vi "initialize NI card.vi"(7 "do waveforms":T5[](array[typedef]), 11 "error in":errorcluster) -> (4 "main trigger":refnum<k21>, 15 "error out":errorcluster)   [LabVIEW 2015]
uses:
  type def/NI card channels.ctl
  type def/do waveform.ctl
  type def/basic params.ctl
  type def/advanced params.ctl
  type def/PXI control.ctl
  <instrlib>/niScope/Controls/niScope trigger source digital.ctl
  <instrlib>/niScope/Controls/niScope trigger slope.ctl
  <vilib>/DAQmx/write.llb/DAQmx Write (Digital 1D U32 1Chan NSamp).vi
  global variables/params.vi
  <instrlib>/niScope/Configure/Trigger/niScope Configure Trigger Digital.vi
  <vilib>/DAQmx/create/channels.llb/DAQmx Create Channel (CO-Pulse Generation-Time).vi
  <vilib>/DAQmx/configure/timing.llb/DAQmx Timing (Implicit).vi
  <vilib>/DAQmx/configure/trigger.llb/DAQmx Start Trigger (None).vi
  <vilib>/DAQmx/configure/trigger.llb/DAQmx Start Trigger (Digital Edge).vi
  <vilib>/DAQmx/create/channels.llb/DAQmx Create Channel (CO-Pulse Generation-Frequency).vi
  <vilib>/DAQmx/create/channels.llb/DAQmx Create Channel (DO-Digital Output).vi
  <vilib>/DAQmx/configure/timing.llb/DAQmx Timing (Sample Clock).vi
  <vilib>/DAQmx/miscellaneous.llb/DAQmx Fill In Error Info.vi
  <resource>/objmgr/daqmx.rc
panel:
  in  "PXI channel":T1={"Vertical Range (V)"=1.0, "Min Sample Rate"=2208791.906743315, "# of Channels"=1, "Min Record Length"=560, "Number Of Records"=10000, "Trigger Position(%)"=0.0, "act Record Length"=1000, "trigger source"="VAL_EXTERNAL", "PMT2 # of Channels"=1} {"PMT2 # of Channels" min=1 max=8 step=1; "act Record Length" min=0 max=100 format="%#.3g"; "Trigger Position(%)" min=0.0 max=1000000.0 step=1.0 format="%#.3p"; "Number Of Records" min=0 max=10000 step=1 format="%#.3g"; "Min Record Length" min=1 max=8 step=1; "# of Channels" min=1 max=8 step=1; "Min Sample Rate" min=0.0 max=100000000.0 format="%#.3p"; "Vertical Range (V)" min=0.0 max=10.0 format="%#.3g"}
  in  "advanced params":T3={"x flyback time(%)"=40.0, "signal offset"=0, "frame time(s)"=0.0, "fetch # per frame"=1, "galvo sampling rate"=500000} {"galvo sampling rate" min=10000 max=200000 step=1; "fetch # per frame" min=1 max=100 step=1 format="%#.3g"; "frame time(s)" min=0.0 max=100.0 step=0.1 format="%#.3g"; "signal offset" max=10000 format="%#.3g"; "x flyback time(%)" min=0.0 max=50.0 format="%#.3g"}
  in  "basic params":T4={"X pixel #"=200, "X pixel size(um)"=1.0, "Y pixel #"=200, "Y pixel size(um)"=10.0, "line rate(Hz)"=1.0, "stage scan?"=FALSE} {"line rate(Hz)" min=1.0 max=2000.0 format="%#.3g"; "X pixel size(um)" min=0.0 max=10.0 format="%#.3g"; "X pixel #" min=2 max=20480 step=2 format="%#.3g"; "Y pixel size(um)" min=0.0 max=10.0 format="%#.3g"; "Y pixel #" min=2 max=204800 step=2 format="%#.3g"}
  in  "do":T6=[{"signal"="x galvo", "DAQmx Physical Channel"="Dev1/ao0", "max"=10.0, "min"=-10.0, "DAQmx Terminal"="", "start trigger"="", "ClockSource"="", "Scaling Factor"=1.0, "Notes"=""}, {"signal"="y galvo", "DAQmx Physical Channel"="Dev1/ao1", "max"=10.0, "min"=-10.0, "DAQmx Terminal"="", "start trigger"="", "ClockSource"="", "Scaling Factor"=1.0, "Notes"=""}]
  in  "triggers":T6=[{"signal"="x galvo", "DAQmx Physical Channel"="Dev1/ao0", "max"=10.0, "min"=-10.0, "DAQmx Terminal"="", "start trigger"="", "ClockSource"="", "Scaling Factor"=1.0, "Notes"=""}, {"signal"="y galvo", "DAQmx Physical Channel"="Dev1/ao1", "max"=10.0, "min"=-10.0, "DAQmx Terminal"="", "start trigger"="", "ClockSource"="", "Scaling Factor"=1.0, "Notes"=""}]
  in  "NI card channels":T6=[{"signal"="x galvo", "DAQmx Physical Channel"="Dev1/ao0", "max"=10.0, "min"=-10.0, "DAQmx Terminal"="", "start trigger"="", "ClockSource"="", "Scaling Factor"=1.0, "Notes"=""}, {"signal"="y galvo", "DAQmx Physical Channel"="Dev1/ao1", "max"=10.0, "min"=-10.0, "DAQmx Terminal"="", "start trigger"="", "ClockSource"="", "Scaling Factor"=1.0, "Notes"=""}]
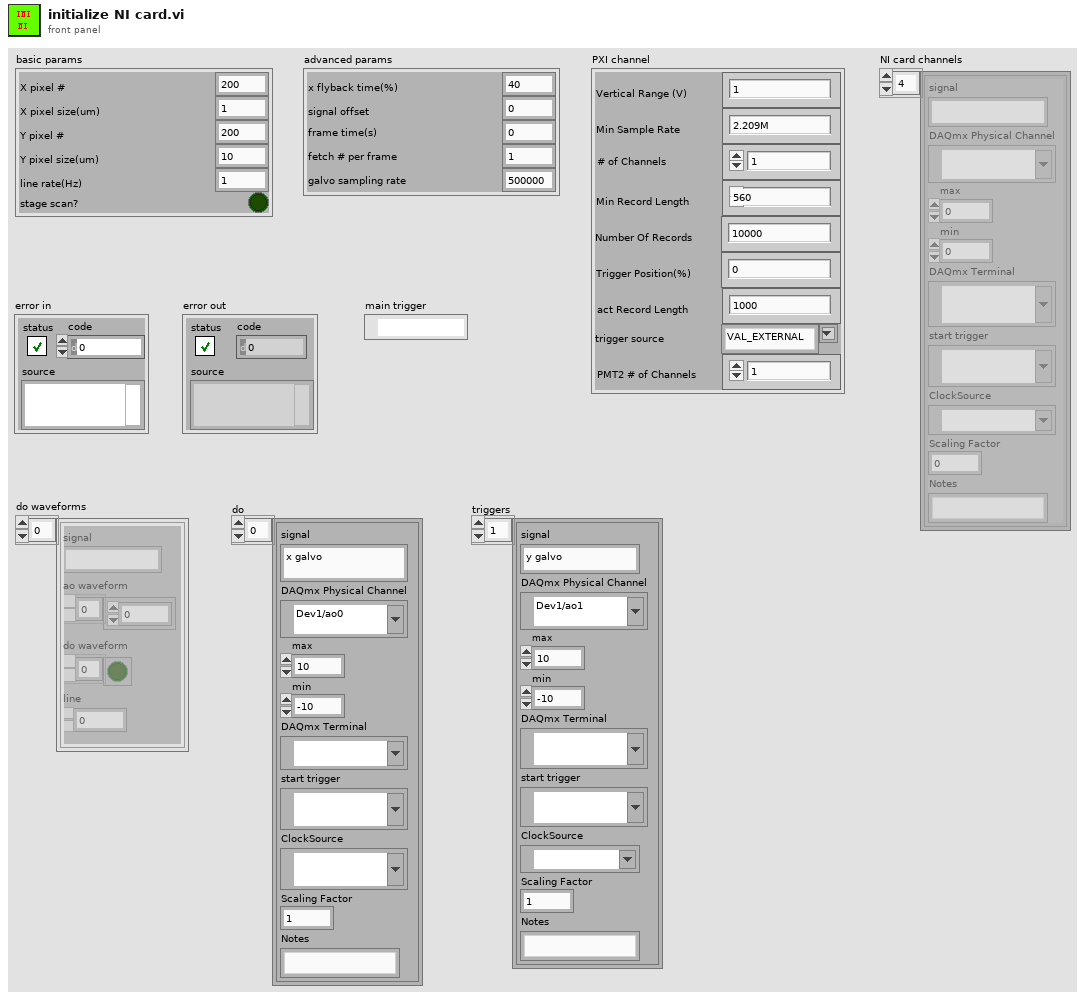
[diagram p1: front panel]
types:
  T1 = typedef "PXI control.ctl" = cluster{"Vertical Range (V)":dbl, "Min Sample Rate":dbl, "# of Channels":u8, "Min Record Length":i32, "Number Of Records":i32, "Trigger Position(%)":dbl, "act Record Length":i32, "trigger source":T2, "PMT2 # of Channels":u8}
  T2 = typedef "niScope trigger source digital.ctl" = string
  T3 = typedef "advanced params.ctl" = cluster{"x flyback time(%)":dbl, "signal offset":u16, "frame time(s)":dbl, "fetch # per frame":u16, "galvo sampling rate":u32}
  T4 = typedef "basic params.ctl" = cluster{"X pixel #":u32, "X pixel size(um)":dbl, "Y pixel #":u32, "Y pixel size(um)":dbl, "line rate(Hz)":dbl, "stage scan?":bool}
  T5 = typedef "do waveform.ctl" = cluster{"signal":string, "ao waveform":dbl[], "do waveform":bool[], "line":u8}
  T6 = typedef "NI card channels.ctl" = cluster{"signal":string, "DAQmx Physical Channel":tag, "max":dbl, "min":dbl, "DAQmx Terminal":tag, "start trigger":tag, "ClockSource":tag, "Scaling Factor":dbl, "Notes":string}[]
  T7 = cluster{"signal":string, "DAQmx Physical Channel":tag, "max":dbl, "min":dbl, "DAQmx Terminal":tag, "start trigger":string, "ClockSource":tag, "Scaling Factor":dbl, "Notes":string}[]
  T8 = typedef "niScope trigger slope.ctl" = i32
  T9 = typedef "NI tasks.ctl" = cluster{"frame trigger":refnum<k21>, "do":refnum<k21>, "digital galvo clock":refnum<k21>, "PMT in":refnum<k15>, "PMT2 in":refnum<k15>}
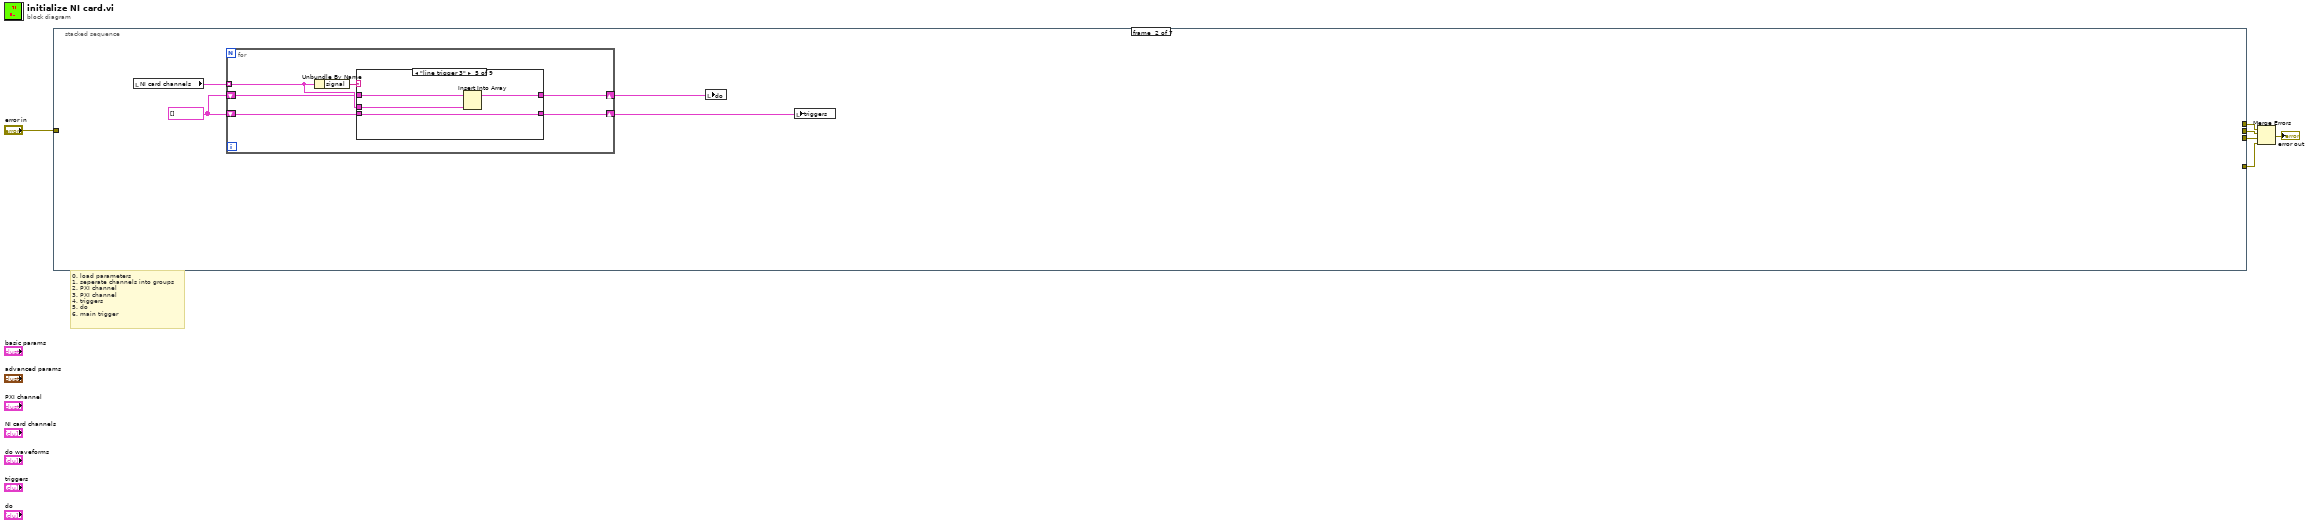
[diagram p0: block diagram]
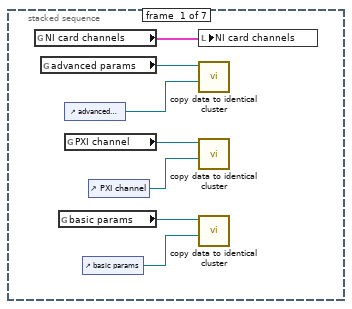
[diagram p2: hidden frame]
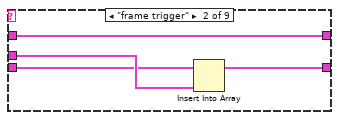
[diagram p4: hidden frame]
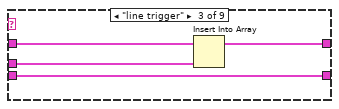
[diagram p5: hidden frame]
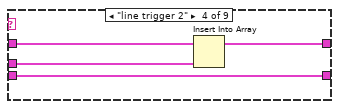
[diagram p6: hidden frame]
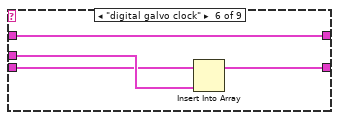
[diagram p7: hidden frame]
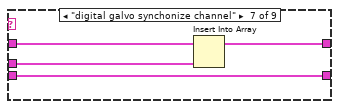
[diagram p8: hidden frame]
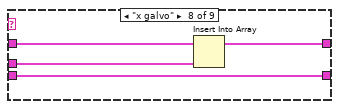
[diagram p9: hidden frame]
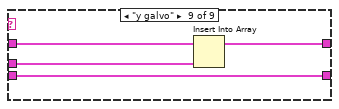
[diagram p10: hidden frame]
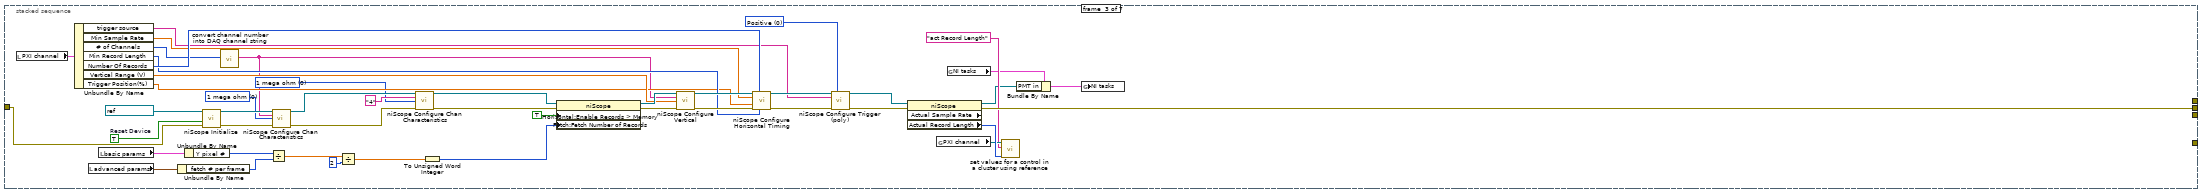
[diagram p11: hidden frame]
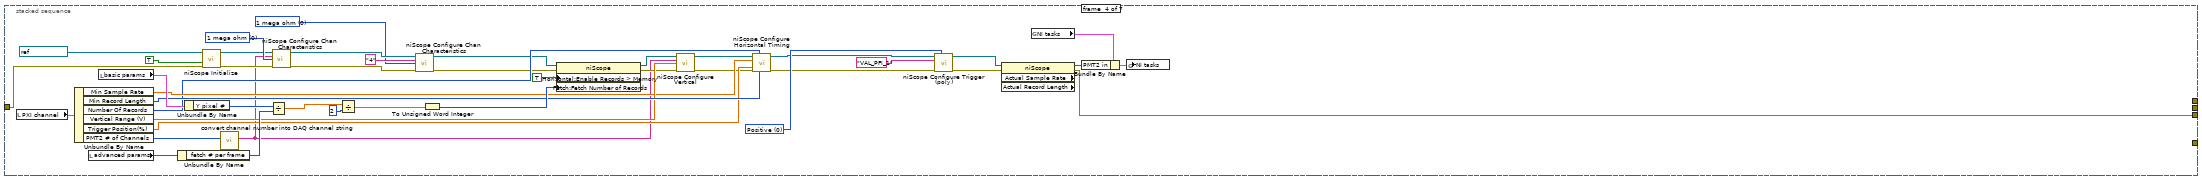
[diagram p12: hidden frame]
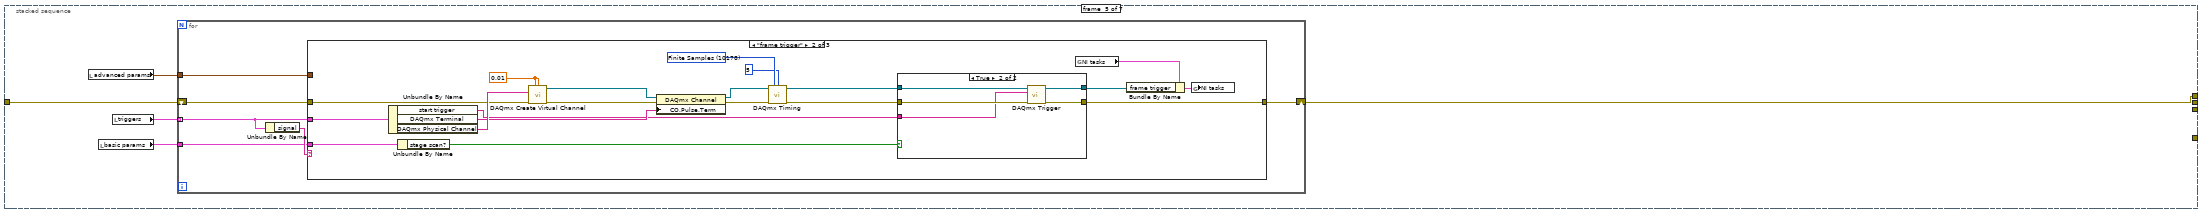
[diagram p13: hidden frame]
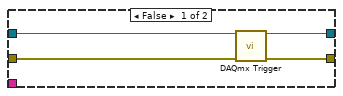
[diagram p15: hidden frame]
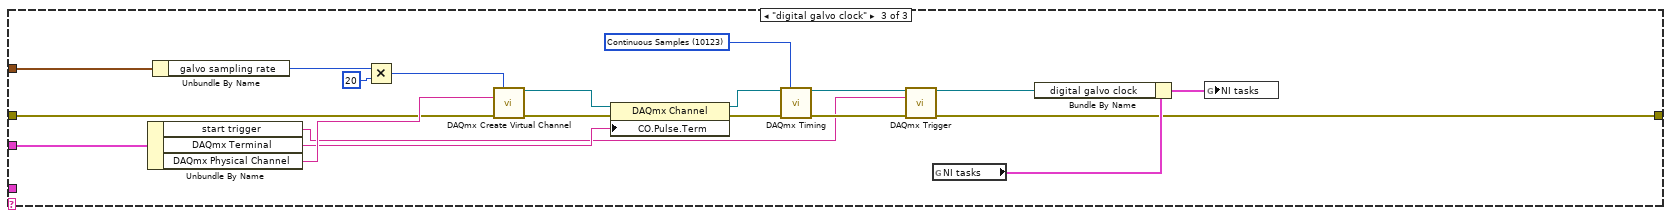
[diagram p16: hidden frame]
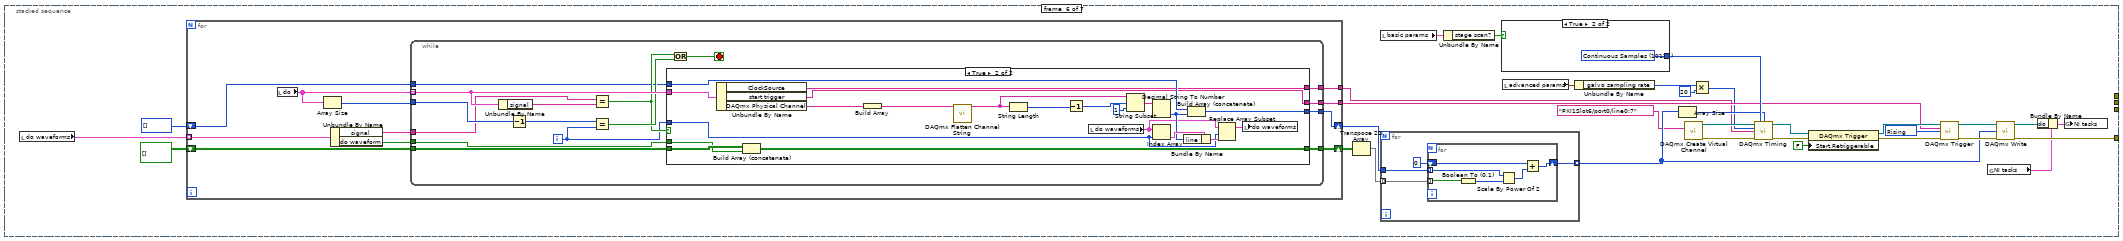
[diagram p17: hidden frame]
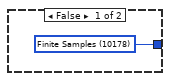
[diagram p18: hidden frame]
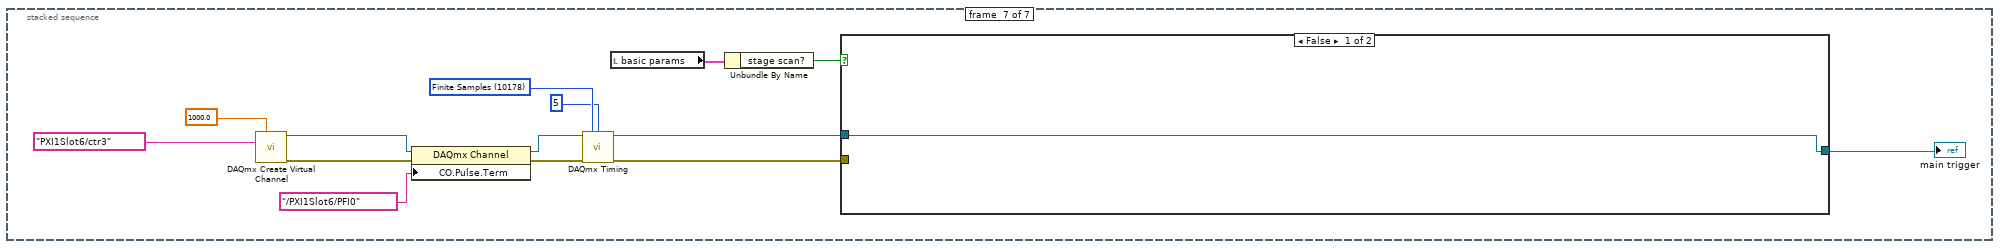
[diagram p20: hidden frame]
diagram:
  # "0. load parameters\n1. seperate channels into groups\n2. PXI channel\n3. PXI channel\n4. triggers\n5. do\n6. main trigger"
  n1 = stacked-sequence {
    tunnel: "error in" -> [_ _ w97 w118 w150 _ _]
    tunnel: [_ _ w87 _ _ _ _] -> w2
    tunnel: [_ _ _ _ w149 _ _] -> w3
    tunnel: [_ _ _ _ _ w227 _] -> w4
    tunnel: [_ _ _ w114 _ _ _] -> w1
    frame #0 {
      n2 = global read "params.vi" "NI card channels"() -> (w12:T6)
      n3 = global read "params.vi" "advanced params"() -> (w13:refnum<vi>)
      n4 = global read "params.vi" "basic params"() -> (w11:refnum<vi>)
      n5 = control-ref of="advanced params"() -> (w8:refnum<vi>)
      n6 = global read "params.vi" "PXI channel"() -> (w10:refnum<vi>)
      n7 = control-ref of="basic params"() -> (w9:refnum<vi>)
      n8 = control-ref of="PXI channel"() -> (w7:refnum<vi>)
      n9 = local write "NI card channels"(w12) -> ()
      n10 = call "copy data to identical cluster.vi"("Guest Clust Refnum"=w8, "Host Clust Refnum"=w13) -> ()  [unwired: 10 in]
      n11 = call "copy data to identical cluster.vi"("Guest Clust Refnum"=w7, "Host Clust Refnum"=w10) -> ()  [unwired: 10 in]
      n12 = call "copy data to identical cluster.vi"("Guest Clust Refnum"=w9, "Host Clust Refnum"=w11) -> ()  [unwired: 10 in]
    }
    frame #1 {
      w14 = T7 []
      n13 = local read "NI card channels"() -> (w17:T6)
      n14 = for {
        tunnel: w17 -> [w22] mode=indexing
        shift-right: [w21] -> w16
        shift-left: w14 -> [w18]
        shift-right: [w20] -> w15
        shift-left: w14 -> [w19]
        n15 = Unbundle By Name(w22) -> ("signal"=w23:string)
        n16 = case shown="\"line trigger 3\"" w23 {
          tunnel: w22 -> [_ w29 w33 w37 w41 w45 w49 w53 w57]
          tunnel: [w25 w27 w30 w34 w38 w44 w48 w50 w56] -> w21
          tunnel: w18 -> [w25 w26 w30 w34 w38 w43 w48 w50 w56]
          tunnel: [w24 w28 w32 w36 w40 w42 w46 w52 w54] -> w20
          tunnel: w19 -> [w24 w28 w31 w35 w39 w42 w47 w51 w55]
          frame "False", Default {
          }
          frame "frame trigger" {
            n17 = Insert Into Array(array=w26, new element=w29) -> (w27:T7)  [unwired: 1 in]
          }
          frame "line trigger" {
            n18 = Insert Into Array(array=w31, new element=w33) -> (w32:T7)  [unwired: 1 in]
          }
          frame "line trigger 2" {
            n19 = Insert Into Array(array=w35, new element=w37) -> (w36:T7)  [unwired: 1 in]
          }
          frame "line trigger 3" {
            n20 = Insert Into Array(array=w39, new element=w41) -> (w40:T7)  [unwired: 1 in]
          }
          frame "digital galvo clock" {
            n21 = Insert Into Array(array=w43, new element=w45) -> (w44:T7)  [unwired: 1 in]
          }
          frame "digital galvo synchonize channel" {
            n22 = Insert Into Array(array=w47, new element=w49) -> (w46:T7)  [unwired: 1 in]
          }
          frame "x galvo" {
            n23 = Insert Into Array(array=w51, new element=w53) -> (w52:T7)  [unwired: 1 in]
          }
          frame "y galvo" {
            n24 = Insert Into Array(array=w55, new element=w57) -> (w54:T7)  [unwired: 1 in]
          }
        }
      }
      n25 = local write "do"(w15) -> ()
      n26 = local write "triggers"(w16) -> ()
    }
    frame #2 {
      w58 = u32 0 items=["1 mega ohm"=0, "50 ohms"=2] ("input impedance")
      w66 = u32 0 items=["1 mega ohm"=0, "50 ohms"=2] ("input impedance")
      w77 = T8 0 items=["Positive", "Negative"] ("trigger slope")
      w103 = TRUE  # Reset Device
      n27 = local read "PXI channel"() -> (w96:T1)
      n28 = Unbundle By Name(w96) -> ("trigger source"=w69:T2, "Min Sample Rate"=w89:dbl, "# of Channels"=w70:u8, "Min Record Length"=w86:i32, "Number Of Records"=w98:i32, "Vertical Range (V)"=w68:dbl, "Trigger Position(%)"=w67:dbl)
      n29 = local read "advanced params"() -> (w95:T3)
      n30 = local read "basic params"() -> (w94:T4)
      n31 = Unbundle By Name(w95) -> ("fetch # per frame"=w76:u16)
      n32 = Unbundle By Name(w94) -> ("Y pixel #"=w91:u32)
      n33 = call <instrlib>:"niScope Initialize.vi"("resource name"=refnum<k15> "PXI1Slot2", "reset device"=w103, "error in"=w97) -> ("instrument handle"=w85:refnum<k15>, "error out"=w84:errorcluster)  [unwired: 11 in]
      n34 = call "convert channel number into DAQ channel string.vi"("Numeric"=w70) -> ("String"=w65:string)  [unwired: 10 in]
      n35 = Divide(x=w91, y=w76) -> (x/y=w74:dbl)
      n36 = call <instrlib>:"niScope Configure Chan Characteristics.vi"("instrument handle"=w85, "channels"=w65, "input impedance"=w66, "error in"=w84) -> ("instrument handle out"=w61:refnum<k15>, "error out"=w60:errorcluster)  [unwired: 10 in]
      n37 = Divide(x=w74, y=2) -> (x/y=w73:dbl)
      n38 = call <instrlib>:"niScope Configure Chan Characteristics.vi"("instrument handle"=w61, "channels"="4", "input impedance"=w58, "error in"=w60) -> ("instrument handle out"=w63:refnum<k15>, "error out"=w62:errorcluster)  [unwired: 10 in]
      n39 = To Unsigned Word Integer(number=w73) -> (unsigned 16bit integer=w72:u16)
      n40 = property class="niScope"(reference=w63, error in=w62, "Horizontal:Enable Records > Memory"=TRUE ("Allow More Records\nthan Available Memory?"), "Fetch:Fetch Number of Records"=w72) -> (reference out=w93:refnum<k15>, error out=w92:errorcluster)
      n41 = call <instrlib>:"niScope Configure Vertical.vi"("instrument handle"=w93, "channels"=w65, "vertical range"=w68, "error in"=w92) -> ("instrument handle out"=w101:refnum<k15>, "error out"=w100:errorcluster)  [unwired: 10 in]
      n42 = call <instrlib>:"niScope Configure Horizontal Timing.vi"("instrument handle"=w101, "number of records"=w98, "min sample rate"=w89, "reference position"=w67, "error in"=w100, "min record length"=w86) -> ("instrument handle out"=w71:refnum<k15>, "error out"=w99:errorcluster)  [unwired: 8 in]
      n43 = call-poly <instrlib>:"niScope Configure Trigger (poly).vi"("instrument handle"=w71, "trigger slope"=w77, "trigger source"=w69, "error in"=w99) -> ("instrument handle out"=w90:refnum<k15>, "error out"=w88:errorcluster)  [unwired: 10 in]
      n44 = property class="niScope" props=["Actual Sample Rate", "Actual Record Length"](reference=w90, error in=w88) -> (reference out=w80:refnum<k15>, error out=w87:errorcluster, "Actual Record Length"=w83:i32)  [unwired: 1 out]
      n45 = global read "params.vi" "PXI channel"() -> (w82:refnum<vi>)
      n46 = global read "params.vi" "NI tasks"() -> (w79:T9)
      n47 = call "set values for a control in a cluster using reference.vi"("value"=w83, "name"="act Record Length", "Clust Refnum"=w82) -> ()  [unwired: 9 in]
      n48 = Bundle By Name(cluster=w79, "PMT in"=w80) -> (w78:T9)
      n49 = global write "params.vi" "NI tasks"(w78) -> ()
    }
    frame #3 {
      w104 = u32 0 items=["1 mega ohm"=0, "50 ohms"=2] ("input impedance")
      w133 = T8 0 items=["Positive", "Negative"] ("trigger slope")
      w123 = u32 0 items=["1 mega ohm"=0, "50 ohms"=2] ("input impedance")
      n50 = local read "PXI channel"() -> (w127:T1)
      n51 = Unbundle By Name(w127) -> ("Min Sample Rate"=w135:dbl, "Min Record Length"=w138:i32, "Number Of Records"=w134:i32, "Vertical Range (V)"=w137:dbl, "Trigger Position(%)"=w136:dbl, "PMT2 # of Channels"=w111:u8)
      n52 = local read "advanced params"() -> (w143:T3)
      n53 = local read "basic params"() -> (w145:T4)
      n54 = Unbundle By Name(w143) -> ("fetch # per frame"=w142:u16)
      n55 = Unbundle By Name(w145) -> ("Y pixel #"=w146:u32)
      n56 = call <instrlib>:"niScope Initialize.vi"("resource name"=refnum<k15> "PXI1Slot3", "reset device"=TRUE, "error in"=w118) -> ("instrument handle"=w119:refnum<k15>, "error out"=w120:errorcluster)  [unwired: 11 in]
      n57 = call "convert channel number into DAQ channel string.vi"("Numeric"=w111) -> ("String"=w110:string)  [unwired: 10 in]
      n58 = Divide(x=w146, y=w142) -> (x/y=w140:dbl)
      n59 = call <instrlib>:"niScope Configure Chan Characteristics.vi"("instrument handle"=w119, "channels"=w110, "input impedance"=w123, "error in"=w120) -> ("instrument handle out"=w109:refnum<k15>, "error out"=w108:errorcluster)  [unwired: 10 in]
      n60 = Divide(x=w140, y=2) -> (x/y=w139:dbl)
      n61 = call <instrlib>:"niScope Configure Chan Characteristics.vi"("instrument handle"=w109, "channels"="4", "input impedance"=w104, "error in"=w108) -> ("instrument handle out"=w107:refnum<k15>, "error out"=w106:errorcluster)  [unwired: 10 in]
      n62 = To Unsigned Word Integer(number=w139) -> (unsigned 16bit integer=w144:u16)
      n63 = property class="niScope"(reference=w107, error in=w106, "Horizontal:Enable Records > Memory"=TRUE, "Fetch:Fetch Number of Records"=w144) -> (reference out=w125:refnum<k15>, error out=w126:errorcluster)
      n64 = call <instrlib>:"niScope Configure Vertical.vi"("instrument handle"=w125, "channels"=w110, "vertical range"=w137, "error in"=w126) -> ("instrument handle out"=w129:refnum<k15>, "error out"=w130:errorcluster)  [unwired: 10 in]
      n65 = call <instrlib>:"niScope Configure Horizontal Timing.vi"("instrument handle"=w129, "number of records"=w134, "min sample rate"=w135, "reference position"=w136, "error in"=w130, "min record length"=w138) -> ("instrument handle out"=w128:refnum<k15>, "error out"=w131:errorcluster)  [unwired: 8 in]
      n66 = call-poly <instrlib>:"niScope Configure Trigger (poly).vi"("instrument handle"=w128, "trigger slope"=w133, "trigger source"=T2 "VAL_PFI_1", "error in"=w131) -> ("instrument handle out"=w113:refnum<k15>, "error out"=w115:errorcluster)  [unwired: 10 in]
      n67 = property class="niScope" props=["Actual Sample Rate", "Actual Record Length"](reference=w113, error in=w115) -> (reference out=w112:refnum<k15>, error out=w114:errorcluster)  [unwired: 2 out]
      n68 = global read "params.vi" "NI tasks"() -> (w117:T9)
      n69 = Bundle By Name(cluster=w117, "PMT2 in"=w112) -> (w116:T9)
      n70 = global write "params.vi" "NI tasks"(w116) -> ()
    }
    frame #4 {
      n71 = local read "advanced params"() -> (w147:T3)
      n72 = local read "basic params"() -> (w148:T4)
      n73 = local read "triggers"() -> (w151:T6)
      n74 = for {
        tunnel: w151 -> [w156] mode=indexing
        shift-right: [w155] -> w149
        shift-left: w150 -> [w154]
        tunnel: w148 -> [w153]
        tunnel: w147 -> [w152]
        n75 = Unbundle By Name(w156) -> ("signal"=w157:string)
        n76 = case shown="\"frame trigger\"" w157 {
          tunnel: w156 -> [_ w178 w207]
          tunnel: w154 -> [w158 w170 w200]
          tunnel: [w158 w162 w196] -> w155
          tunnel: w153 -> [_ w159 _]
          tunnel: w152 -> [_ _ w192]
          frame "False", Default {
          }
          frame "frame trigger" {
            w167 = 0.01 ("high time")
            w171 = 10178 items=["Finite Samples"=10178, "Continuous Samples"=10123, "Hardware Timed Single Point"=12522] ("sample mode")
            n77 = Unbundle By Name(w178) -> ("start trigger"=w160:tag, "DAQmx Terminal"=w174:tag, "DAQmx Physical Channel"=w175:tag)
            n78 = Unbundle By Name(w159) -> ("stage scan?"=w161:bool)
            n79 = call-poly <vilib>:"DAQmx Create Virtual Channel.vi"("high time"=w167, "low time"=w167, "counter"=w175, "error in"=w170) -> ("task out"=w176:refnum<k21>, "error out"=w177:errorcluster)  [unwired: 10 in]
            n80 = property class="DAQmx Channel"(reference=w176, error in=w177, "CO.Pulse.Term"=w174) -> (reference out=w173:refnum<k21>, error out=w172:errorcluster)
            n81 = call-poly <vilib>:"DAQmx Timing.vi"("task/channels in"=w173, "sample mode"=w171, "samples per channel"=5, "error in"=w172) -> ("task out"=w165:refnum<k21>, "error out"=w163:errorcluster)  [unwired: 10 in]
            n82 = case shown="True" w161 {
              tunnel: w165 -> [w182 w187]
              tunnel: [w181 w186] -> w164
              tunnel: w163 -> [w180 w185]
              tunnel: [w179 w184] -> w162
              tunnel: w160 -> [_ w183]
              frame False {
                n83 = call-poly <vilib>:"DAQmx Trigger.vi"("task/channels in"=w182, "error in"=w180) -> ("task out"=w181:refnum<k21>, "error out"=w179:errorcluster)  [unwired: 12 in]
              }
              frame True {
                n84 = call-poly <vilib>:"DAQmx Trigger.vi"("task/channels in"=w187, "source"=w183, "error in"=w185) -> ("task out"=w186:refnum<k21>, "error out"=w184:errorcluster)  [unwired: 11 in]
              }
            }
            n85 = global read "params.vi" "NI tasks"() -> (w169:T9)
            n86 = Bundle By Name(cluster=w169, "frame trigger"=w164) -> (w168:T9)
            n87 = global write "params.vi" "NI tasks"(w168) -> ()
          }
          frame "digital galvo clock" {
            w195 = 10123 items=["Finite Samples"=10178, "Continuous Samples"=10123, "Hardware Timed Single Point"=12522] ("sample mode")
            n88 = Unbundle By Name(w207) -> ("start trigger"=w188:tag, "DAQmx Terminal"=w203:tag, "DAQmx Physical Channel"=w204:tag)
            n89 = Unbundle By Name(w192) -> ("galvo sampling rate"=w191:u32)
            n90 = Multiply(x=w191, y=u32 20) -> (x*y=w189:u32)
            n91 = call-poly <vilib>:"DAQmx Create Virtual Channel.vi"("frequency"=w189, "counter"=w204, "error in"=w200) -> ("task out"=w205:refnum<k21>, "error out"=w206:errorcluster)  [unwired: 11 in]
            n92 = property class="DAQmx Channel"(reference=w205, error in=w206, "CO.Pulse.Term"=w203) -> (reference out=w202:refnum<k21>, error out=w201:errorcluster)
            n93 = call-poly <vilib>:"DAQmx Timing.vi"("task/channels in"=w202, "sample mode"=w195, "error in"=w201) -> ("task out"=w194:refnum<k21>, "error out"=w193:errorcluster)  [unwired: 11 in]
            n94 = call-poly <vilib>:"DAQmx Trigger.vi"("task/channels in"=w194, "source"=w188, "error in"=w193) -> ("task out"=w197:refnum<k21>, "error out"=w196:errorcluster)  [unwired: 11 in]
            n95 = global read "params.vi" "NI tasks"() -> (w199:T9)
            n96 = Bundle By Name(cluster=w199, "digital galvo clock"=w197) -> (w198:T9)
            n97 = global write "params.vi" "NI tasks"(w198) -> ()
          }
        }
      }
    }
    frame #5 {
      w221 = 10280 items=["Rising"=10280, "Falling"=10171] ("edge")
      n98 = local read "do waveforms"() -> (w235:T5[])
      n99 = for {
        tunnel: w235 -> [w249] mode=indexing
        shift-right: [w248] -> w234
        shift-left: bool[][] [] -> [w247]
        shift-right: [w246] -> w237
        shift-left: i32[] [] -> [w245]
        tunnel: [w244] -> w216
        tunnel: [w242] -> w215
        n100 = local read "do"() -> (w243:T6)
        n101 = Array Size(array=w243) -> (size(s)=w251:i32)
        n102 = Unbundle By Name(w249) -> ("signal"=w252:string, "do waveform"=w250:bool[])
        n103 = while {
          tunnel: w243 -> [w268] mode=indexing
          tunnel: w252 -> [w254]
          tunnel: w251 -> [w267]
          tunnel: w250 -> [w262]
          tunnel: [w261] -> w248
          tunnel: w247 -> [w260]
          tunnel: w245 -> [w259]
          tunnel: [w258] -> w246
          tunnel: [w257] -> w244
          tunnel: [w253] -> w242
          i -> [w256]
          stop <- w263 stop-if-true
          n104 = Unbundle By Name(w268) -> ("signal"=w255:string)
          n105 = Decrement(x=w267) -> (x-1=w266:i32)
          n106 = Equal?(x=w254, y=w255) -> (x = y?=w264:bool)
          n107 = Equal?(x=w266, y=w256) -> (x = y?=w265:bool)
          n108 = case shown="True" w264 {
            tunnel: w268 -> [_ w291]
            tunnel: w262 -> [_ w288]
            tunnel: [w270 w290] -> w261
            tunnel: w260 -> [w270 w289]
            tunnel: w259 -> [w269 w280]
            tunnel: [w269 w279] -> w258
            tunnel: [_ w278] -> w257
            tunnel: w256 -> [_ w274]
            tunnel: [_ w271] -> w253
            frame False {
            }
            frame True {
              n109 = Unbundle By Name(w291) -> ("ClockSource"=w271:tag, "start trigger"=w278:tag, "DAQmx Physical Channel"=w287:tag)
              n110 = Build Array (concatenate)(w289, w288) -> (w290:bool[][])
              n111 = Build Array(w287) -> (w286:tag[])
              n112 = call <vilib>:"DAQmx Flatten Channel String.vi"("names in"=w286) -> ("names out"=w282:string)  [unwired: 13 in, 1 out]
              n113 = String Length(string=w282) -> (length=w283:i32)
              n114 = Decrement(x=w283) -> (x-1=w284:i32)
              n115 = local read "do waveforms"() -> (w272:T5[])
              n116 = String Subset(string=w282, offset (0)=w284, length (rest)=1 ("length (rest)")) -> (substring=w281:string)
              n117 = Decimal String To Number(string=w281) -> (number=w276:i32)  [unwired: 2 in, 1 out]
              n118 = Index Array(array=w272, index=w274) -> (element=w277:T5)
              n119 = Bundle By Name(cluster=w277, "line"=w276) -> (w275:T5)
              n120 = Build Array (concatenate)(w280, w276) -> (w279:i32[])
              n121 = Replace Array Subset(array=w272, new element=w275, index=w274) -> (w273:T5[])
              n122 = local write "do waveforms"(w273) -> ()
            }
          }
          n123 = Or(x=w264, y=w265) -> (x .or. y?=w263:bool)
        }
      }
      n124 = Transpose 2D Array(2D array=w234) -> (transposed array=w239:bool[][])
      n125 = local read "basic params"() -> (w214:T4)
      n126 = for {
        tunnel: w239 -> [w294] mode=indexing
        tunnel: w237 -> [w295]
        tunnel: [w292] -> w222 mode=indexing
        n127 = for {
          tunnel: w295 -> [w301] mode=indexing
          tunnel: w294 -> [w300] mode=indexing
          shift-right: [w296] -> w292
          shift-left: u32 0 -> [w297]
          n128 = Boolean To (0,1)(Boolean=w300) -> (0, 1=w299:i16)
          n129 = Scale By Power Of 2(n=w301, x=w299) -> (x*2^n=w298:i16)
          n130 = Add(x=w297, y=w298) -> (x+y=w296:u32)
        }
      }
      n131 = Unbundle By Name(w214) -> ("stage scan?"=w213:bool)
      n132 = case shown="True" w213 {
        tunnel: [w240 w241] -> w233
        frame False {
          w240 = 10178 items=["Finite Samples"=10178, "Continuous Samples"=10123, "Hardware Timed Single Point"=12522] ("sample mode")
        }
        frame True {
          w241 = 10123 items=["Finite Samples"=10178, "Continuous Samples"=10123, "Hardware Timed Single Point"=12522] ("sample mode")
        }
      }
      n133 = local read "advanced params"() -> (w211:T3)
      n134 = Unbundle By Name(w211) -> ("galvo sampling rate"=w210:u32)
      n135 = Array Size(array=w222) -> (size(s)=w223:i32)
      n136 = call-poly <vilib>:"DAQmx Create Virtual Channel.vi"("lines"=tag "PXI1Slot6/port0/line0:7" ("Line(s)")) -> ("task out"=w232:refnum<k21>, "error out"=w224:errorcluster)  [unwired: 13 in]
      n137 = Multiply(x=w210, y=u32 20) -> (x*y=w208:u32)
      n138 = call-poly <vilib>:"DAQmx Timing.vi"("task/channels in"=w232, "sample mode"=w233, "samples per channel"=w223, "rate"=w208, "source"=w215, "error in"=w224) -> ("task out"=w226:refnum<k21>, "error out"=w225:errorcluster)  [unwired: 8 in]
      n139 = property class="DAQmx Trigger"(reference=w226, error in=w225, "Start.Retriggerable"=FALSE) -> (reference out=w231:refnum<k21>, error out=w230:errorcluster)
      n140 = call-poly <vilib>:"DAQmx Trigger.vi"("task/channels in"=w231, "source"=w216, "edge"=w221, "error in"=w230) -> ("task out"=w229:refnum<k21>, "error out"=w228:errorcluster)  [unwired: 10 in]
      n141 = global read "params.vi" "NI tasks"() -> (w220:T9)
      n142 = call-poly <vilib>:"DAQmx Write.vi"("task/channels in"=w229, "data"=w222, "error in"=w228) -> ("task out"=w212:refnum<k21>, "error out"=w227:errorcluster)  [unwired: 10 in, 1 out]
      n143 = Bundle By Name(cluster=w220, "do"=w212) -> (w219:T9)
      n144 = global write "params.vi" "NI tasks"(w219) -> ()
    }
    frame #6 {
      w314 = 10178 items=["Finite Samples"=10178, "Continuous Samples"=10123, "Hardware Timed Single Point"=12522] ("sample mode")
      n145 = call-poly <vilib>:"DAQmx Create Virtual Channel.vi"("frequency"=1000.0, "counter"=tag "PXI1Slot6/ctr3") -> ("task out"=w307:refnum<k21>, "error out"=w308:errorcluster)  [unwired: 12 in]
      n146 = property class="DAQmx Channel"(reference=w307, error in=w308, "CO.Pulse.Term"=tag "/PXI1Slot6/PFI0") -> (reference out=w311:refnum<k21>, error out=w312:errorcluster)
      n147 = call-poly <vilib>:"DAQmx Timing.vi"("task/channels in"=w311, "sample mode"=w314, "samples per channel"=5, "error in"=w312) -> ("task out"=w306:refnum<k21>, "error out"=w305:errorcluster)  [unwired: 10 in]
      n148 = local read "basic params"() -> (w303:T4)
      n149 = Unbundle By Name(w303) -> ("stage scan?"=w302:bool)
      n150 = case shown="False" w302 {
        tunnel: w306 -> [w316 w324]
        tunnel: w305 -> [_ w323]
        tunnel: [w316 w317] -> w304
        frame False {
        }
        frame True {
          w321 = 10171 items=["Rising"=10280, "Falling"=10171] ("edge")
          n151 = call-poly <vilib>:"DAQmx Trigger.vi"("task/channels in"=w324, "source"=tag "/PXI1Slot6/PFI12", "edge"=w321, "error in"=w323) -> ("task out"=w319:refnum<k21>, "error out"=w318:errorcluster)  [unwired: 10 in]
          n152 = property class="DAQmx Trigger"(reference=w319, error in=w318, "Start.Retriggerable"=FALSE) -> (reference out=w317:refnum<k21>)  [unwired: 1 out]
        }
      }
      "main trigger" <- w304
    }
  }
  n153 = Merge Errors(w3, w2, w1, w4) -> (→"error out":errorcluster)
